vi "search_video_timestamp.vi"(5 "Status ref":refnum<vi>, 6 "Status prefix":string, 7 "Threads (32)":i32=32, 8 "error in (no error)":errorcluster, 9 "ID rate per day (78k)":i32=78000, 10 "Reference ID record":cluster{"ID":i32, "Time":timestamp}, 11 "Target time":timestamp) -> (0 "error out":errorcluster, 3 "ID at target time":i32)   [LabVIEW 2023]
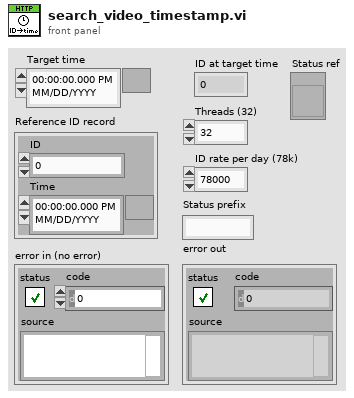
[diagram p1: front panel]
types:
  T1 = cluster{"Status ref":refnum<vi>, "Status prefix":string}
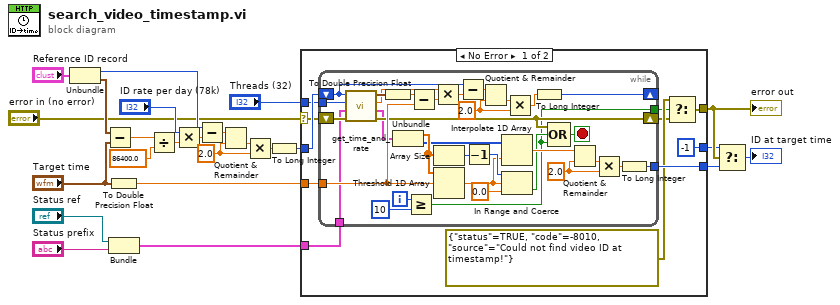
[diagram p0: block diagram]
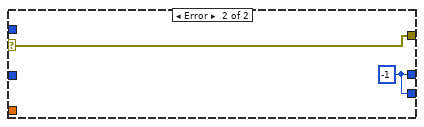
[diagram p2: hidden frame]
diagram:
  w18 = 2.0 ("y")
  n1 = Unbundle("Reference ID record") -> ("ID"=w10:i32, "Time"=w9:timestamp)
  n2 = Subtract(x=w9, y="Target time") -> (x-y=w23:dbl)
  n3 = To Double Precision Float(number="Target time") -> (double precision float=w15:dbl)
  n4 = Bundle("Status ref"="Status ref", "Status prefix"="Status prefix") -> (w1:T1)  [unwired: 1 in]
  n5 = Divide(x=w23, y=86400.0) -> (x/y=w22:dbl)
  n6 = Multiply(x="ID rate per day (78k)", y=w22) -> (x*y=w14:dbl)
  n7 = Subtract(x=w10, y=w14) -> (x-y=w19:dbl)
  n8 = Quotient & Remainder(x=w19, y=w18) -> (floor(x/y)=w17:dbl)  [unwired: 1 out]
  n9 = Multiply(x=w17, y=w18) -> (x*y=w13:dbl)
  n10 = To Long Integer(number=w13) -> (32bit integer=w12:i32)
  n11 = case shown="No Error" "error in (no error)" {
    selector: "error in (no error)" -> [w34 w70]
    tunnel: "Threads (32)" -> [w33 _]
    tunnel: [w28 w70] -> w7
    tunnel: w12 -> [w35 _]
    tunnel: w15 -> [w32 _]
    tunnel: [w31 w69] -> w6
    tunnel: [-1 w69] -> w4
    tunnel: w1 -> [w25 _]
    frame No Error {
      n12 = while {
        tunnel: w33 -> [w67]
        shift-right: [w46] -> w29
        shift-left: w34 -> [w68]
        shift-right: [w48] -> _
        shift-left: w35 -> [w53]
        tunnel: w32 -> [w56]
        tunnel: [w58] -> w31
        tunnel: [w37] -> w27
        tunnel: w25 -> [w36]
        i -> [w39]
        stop <- w44 stop-if-true
        w51 = 2.0 ("y")
        w61 = 2.0 ("y")
        n13 = call "get_time_and_rate.vi"("error in (no error)"=w68, "Status"=w36, "Threads (32)"=w67, "ID"=w53) -> ("error out"=w46:errorcluster, "Scan result"=w43:cluster{"Time (DBL)":dbl[], "Video ID":i32[]}, "ID rate (per second)"=w40:dbl, "ID timestamp"=w47:timestamp)  [unwired: 4 in]
        n14 = To Double Precision Float(number=w47) -> (double precision float=w57:dbl)
        n15 = Unbundle(w43) -> ("Time (DBL)"=w42:dbl[], "Video ID"=w41:i32[])
        n16 = Greater Or Equal?(x=w39, y=10) -> (x >= y?=w37:bool)
        n17 = Subtract(x=w57, y=w56) -> (x-y=w55:dbl)
        n18 = Multiply(x=w40, y=w55) -> (x*y=w54:dbl)
        n19 = Array Size(array=w42) -> (size(s)=w66:i32)
        n20 = Threshold 1D Array(2:w56, 3:w42) -> (0:w63:dbl)  [unwired: 1 in]
        n21 = Subtract(x=w53, y=w54) -> (x-y=w49:dbl)
        n22 = Decrement(x=w66) -> (x-1=w64:i32)
        n23 = Quotient & Remainder(x=w49, y=w51) -> (floor(x/y)=w50:dbl)  [unwired: 1 out]
        n24 = Interpolate 1D Array(1:w63, 2:w41) -> (0:w60:dbl)
        n25 = In Range and Coerce(upper limit=w64, x=w63, lower limit=0.0) -> (In Range?=w45:bool)  [unwired: 1 out]
        n26 = Multiply(x=w50, y=w51) -> (x*y=w52:dbl)
        n27 = To Long Integer(number=w52) -> (32bit integer=w48:i32)
        n28 = Compound Arithmetic op=OR(w46, w45, w37) -> (w44:bool)
        n29 = Quotient & Remainder(x=w60, y=w61) -> (floor(x/y)=w62:dbl)  [unwired: 1 out]
        n30 = Multiply(x=w62, y=w61) -> (x*y=w59:dbl)
        n31 = To Long Integer(number=w59) -> (32bit integer=w58:i32)
      }
      n32 = Select(t=errorcluster {"status"=TRUE, "code"=-8010, "source"="Could not find video ID at timestamp!"} ("error constant"), s=w27, f=w29) -> (s? t:f=w28:errorcluster)
    }
    frame Error {
      w69 = -1
    }
  }
  "error out" <- w7
  n33 = Select(t=w4, s=w7, f=w6) -> (s? t:f=→"ID at target time":i32)
